vi "PID.vi"(0 "Medida":dbl(slide) scale=0.0..2.0, 2 "Referencia":dbl(slide) scale=0.0..2.0, 4 "Kd":dbl(slide) scale=0.0..10.0, 5 "Ki":dbl(slide) scale=0.0..10.0, 6 "Kp":dbl(slide) scale=0.0..10.0) -> (1 "Salida PID (%)":dbl, 3 "T":dbl)   [LabVIEW 2011]
panel:
  out "Salida PID":dbl(graph)
  in  "Límite Inferior":dbl
  in  "Límite Superior":dbl
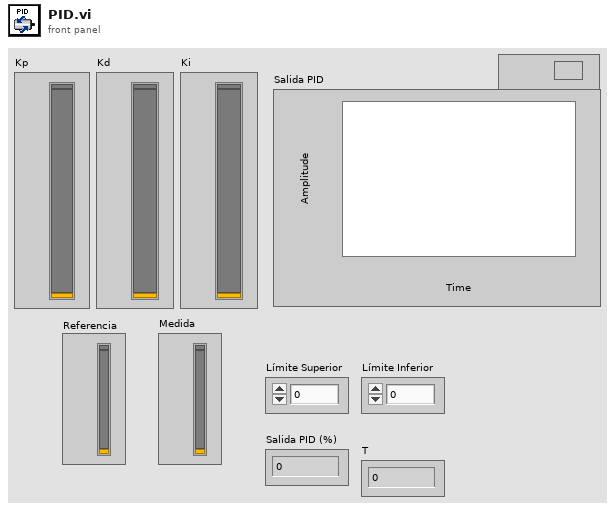
[diagram p1: front panel]
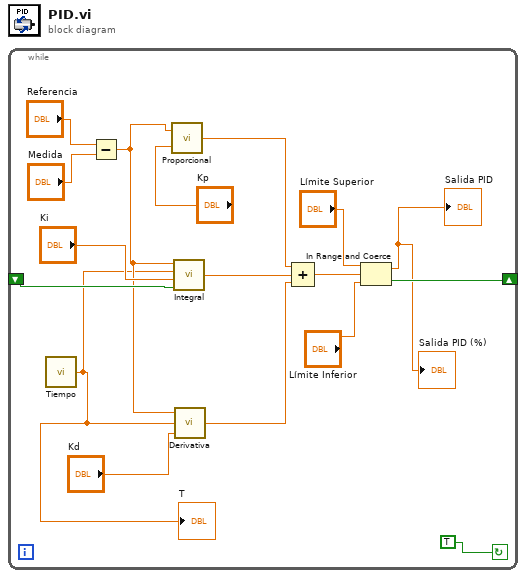
[diagram p0: block diagram]
diagram:
  n1 = while {
    shift-right: [w2] -> _
    shift-left: _ -> [w13]
    stop <- TRUE continue-if-true
    n2 = call "Tiempo.vi"() -> ("Dt"=w9:dbl)
    "T" <- w9
    n3 = Subtract(x="Referencia", y="Medida") -> (x-y=w11:dbl)
    n4 = call "Proporcional.vi"("Kp"="Kp", "Error"=w11) -> ("Acción Proporcional"=w6:dbl)
    n5 = call "Integral.vi"("En rango?"=w13, "KI"="Ki", "Dt"=w9, "Error"=w11) -> ("Acción Integral"=w8:dbl)
    n6 = call "Derivativa.vi"("Kd"="Kd", "Dt"=w9, "Valor Anterior"=w11) -> ("Acción derivativa"=w7:dbl)
    n7 = Compound Arithmetic op=ADD(w6, w8, w7) -> (w5:dbl)
    n8 = In Range and Coerce(upper limit="Límite Superior", x=w5, lower limit="Límite Inferior") -> (coerced(x)=→"Salida PID (%)" →"Salida PID":dbl, In Range?=w2:bool)
  }
